vi "Demo.vi"() -> ()   [LabVIEW 2013]
uses:
  Milk/Milk.lvclass
  Mocha/Mocha.lvclass
  Soy/Soy.lvclass
  Whip/Whip.lvclass
  DarkRoast/DarkRoast.lvclass
  Decaf/Decaf.lvclass
  Espresso/Espresso.lvclass
  CondimentDecorator/CondimentDecorator.lvclass
panel:
  out "OrderList":string
  out "TotalCost":dbl
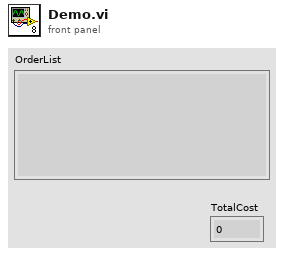
[diagram p1: front panel]
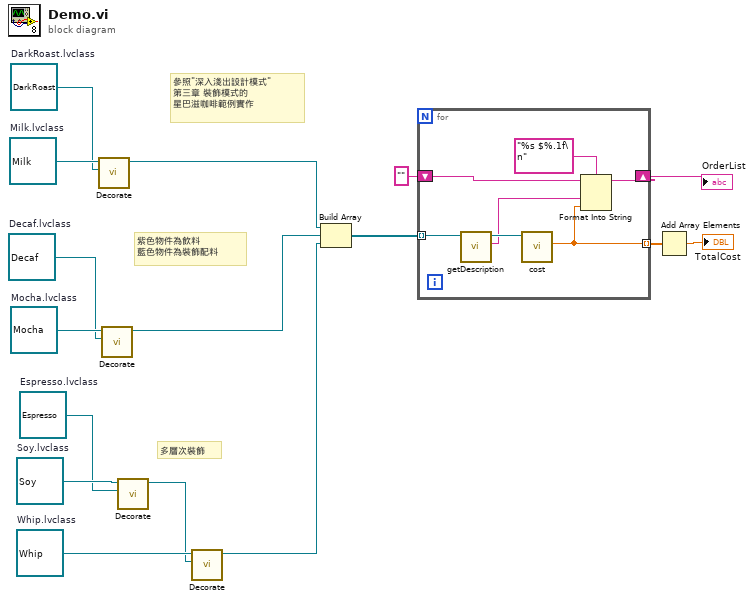
[diagram p0: block diagram]
diagram:
  w9 = refnum<class "Espresso.lvclass"> refnum  # Espresso.lvclass
  w10 = refnum<class "Decaf.lvclass"> refnum  # Decaf.lvclass
  w11 = refnum<class "DarkRoast.lvclass"> refnum  # DarkRoast.lvclass
  w13 = refnum<class "Whip.lvclass"> refnum  # Whip.lvclass
  w14 = refnum<class "Soy.lvclass"> refnum  # Soy.lvclass
  w15 = refnum<class "Mocha.lvclass"> refnum  # Mocha.lvclass
  w16 = refnum<class "Milk.lvclass"> refnum  # Milk.lvclass
  # "多層次裝飾"
  # "紫色物件為飲料\n藍色物件為裝飾配料"
  # "參照\"深入淺出設計模式\"\n第三章 裝飾模式的\n星巴滋咖啡範例實作"
  n1 = call-dynamic "Decorate.vi"("Beverage.lvclass"=w11, "Milk in"=w16) -> ("Milk out"=w8:refnum<class "Milk.lvclass">)  [unwired: 8 in, 1 out]
  n2 = call-dynamic "Decorate.vi"("Beverage.lvclass"=w10, "Mocha in"=w15) -> ("Mocha out"=w7:refnum<class "Mocha.lvclass">)  [unwired: 8 in, 1 out]
  n3 = call-dynamic "Decorate.vi"("Beverage.lvclass"=w9, "Soy in"=w14) -> ("Soy out"=w12:refnum<class "Soy.lvclass">)  [unwired: 8 in, 1 out]
  n4 = call-dynamic "Decorate.vi"("Beverage.lvclass"=w12, "Whip in"=w13) -> ("Whip out"=w6:refnum<class "Whip.lvclass">)  [unwired: 8 in, 1 out]
  n5 = Build Array(w8, w7, w6) -> (w5:refnum<class "CondimentDecorator.lvclass">[])
  n6 = for {
    tunnel: w5 -> [w20] mode=indexing
    shift-right: [w18] -> w4
    shift-left: "" -> [w19]
    tunnel: [w17] -> w3 mode=indexing
    n7 = call-dynamic "getDescription.vi"("Beverage in"=w20) -> ("description"=w22:string, "Beverage out"=w23:refnum<class "CondimentDecorator.lvclass">)  [unwired: 8 in, 1 out]
    n8 = call-dynamic "cost.vi"("Beverage in"=w23) -> ("Cost"=w17:dbl)  [unwired: 8 in, 2 out]
    n9 = Format Into String(format string="%s $%.1f\n", initial string=w19, w22, w17) -> (resulting string=w18:string)  [unwired: 1 in, 1 out]
  }
  "OrderList" <- w4
  n10 = Add Array Elements(numeric array=w3) -> (sum=→"TotalCost":dbl)
